vi "Test Invalid Registration - No Channels Added.vi"() -> ()   [LabVIEW 2024]
uses:
  Mock Sift Proxy Server/Mock Sift Proxy Server.lvclass
  Sift API/Sift Client.lvclass
panel:
  out "Server Error":errorcluster
  out "Success":bool
  out "Error":errorcluster
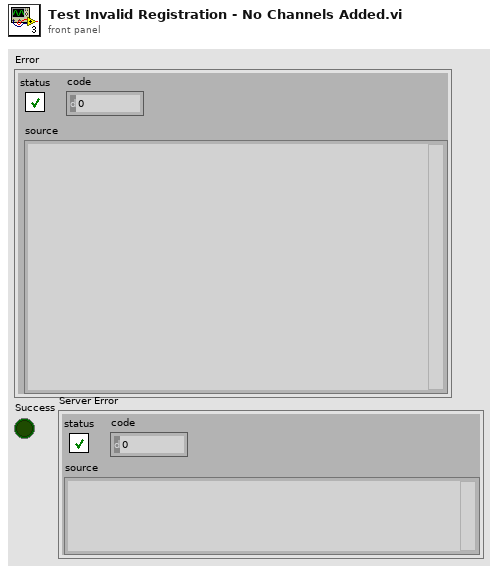
[diagram p1: front panel]
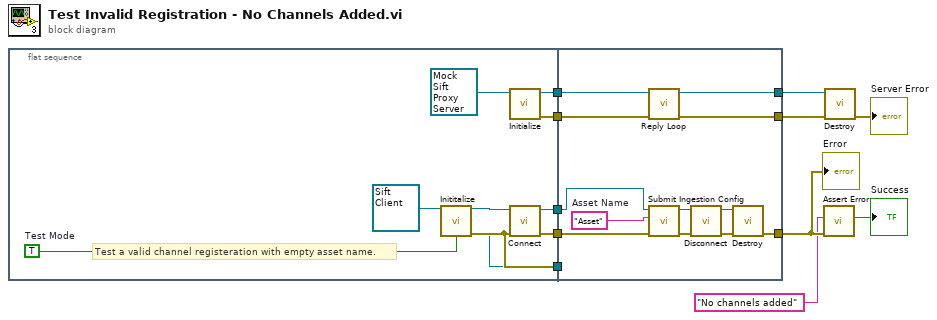
[diagram p0: block diagram]
diagram:
  n1 = flat-sequence {
    tunnel: [w20] -> w12
    tunnel: [w17] -> w11
    tunnel: [w16] -> w10
    tunnel: [w15] -> w9
    tunnel: [w14] -> w8
    tunnel: [w13] -> w7
    tunnel: [w28] -> w5
    tunnel: w12 -> [w29]
    tunnel: [w32] -> w4
    tunnel: w11 -> [_]
    tunnel: w10 -> [_]
    tunnel: w9 -> [w27]
    tunnel: w8 -> [w26]
    tunnel: w7 -> [w23]
    tunnel: [w22] -> w3
    frame #0 {
      w18 = TRUE  # Test Mode
      # "Test a valid channel registeration with empty asset name."
      n2 = call-dynamic "Inititalize.vi"("Sift Client in"=refnum<class "Sift Client.lvclass"> refnum ("Sift Client.lvlib:Sift Client.lvclass"), "Test Mode"=w18) -> ("Sift Client out"=w16:refnum<class "Sift Client.lvclass">, "error out"=w17:errorcluster)  [unwired: 12 in]
      n3 = call-dynamic "Initialize.vi"("Mock Sift Proxy Server in"=refnum<class "Mock Sift Proxy Server.lvclass"> refnum ("Mock Sift Proxy Server.lvclass")) -> ("error out"=w13:errorcluster, "Mock Sift Proxy Server out"=w20:refnum<class "Mock Sift Proxy Server.lvclass">)  [unwired: 9 in]
      n4 = call-dynamic "Connect.vi"("error in (no error)"=w17, "Sift Client in"=w16) -> ("error out"=w15:errorcluster, "Sift Client out"=w14:refnum<class "Sift Client.lvclass">)  [unwired: 7 in, 1 out]
    }
    frame #1 {
      w31 = "Asset"  # Asset Name
      n5 = call-dynamic "Reply Loop.vi"("error in (no error)"=w23, "Mock Sift Proxy Server in"=w29) -> ("error out"=w22:errorcluster, "Mock Sift Proxy Server out"=w28:refnum<class "Mock Sift Proxy Server.lvclass">)  [unwired: 8 in]
      n6 = call-dynamic "Submit Ingestion Config.vi"("error in (no error)"=w27, "Asset Name"=w31, "Sift Client in"=w26) -> ("error out"=w33:errorcluster, "Sift Client out"=w30:refnum<class "Sift Client.lvclass">)  [unwired: 7 in]
      n7 = call-dynamic "Disconnect.vi"("error in (no error)"=w33, "Sift Client in"=w30) -> ("error out"=w24:errorcluster, "Sift Client out"=w25:refnum<class "Sift Client.lvclass">)  [unwired: 8 in]
      n8 = call-dynamic "Destroy.vi"("error in (no error)"=w24, "Sift Client in"=w25) -> ("error out"=w32:errorcluster)  [unwired: 8 in, 1 out]
    }
  }
  n9 = call "Assert Error.vi"("Error"=w4, "Error String"="No channels added") -> ("Success"=→"Success":bool)  [unwired: 9 in]
  n10 = call-dynamic "Destroy.vi"("error in (no error)"=w3, "Mock Sift Proxy Server in"=w5) -> ("error out"=→"Server Error":errorcluster)  [unwired: 8 in, 1 out]
  "Error" <- w4
